vi "modbus type array.vi"() -> (3 "Array":T1[](array[typedef]))   [LabVIEW 2021, in "Modbus Master Shared.lvlib"]
uses:
  Shared/Modbus Master Shared.lvlib
  System Explorer/SubVIs/Modbus Type.ctl
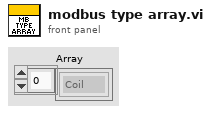
[diagram p1: front panel]
types:
  T1 = typedef "Modbus Master Shared.lvlib/Modbus Type.ctl" = enum16{"Coil", "Discrete Input", "Holding Register", "Input Register"}
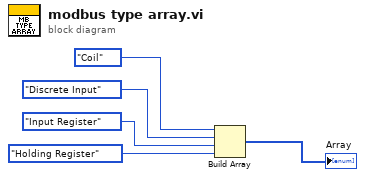
[diagram p0: block diagram]
diagram:
  n1 = Build Array(Modbus_Type."Coil" ("input 1"), Modbus_Type."Discrete Input" ("input 1"), Modbus_Type."Input Register" ("input 1"), Modbus_Type."Holding Register" ("input 1")) -> (→"Array":T1[])
